vi "未命名 13.vi"() -> ()   [LabVIEW 2020]
uses:
  <vilib>/JDP Science/JSONtext/support/Format JSON Object.vi
  <vilib>/JDP Science/JSONtext/JSONtext.lvlib
panel:
  out "<JSON> 2":string[](array[string]) caption="<JSON>Elements"
  out "输出数组":string[](array[string])
  in  "数组":string[](array[string])
  in  "JSON Items":string[](array[string])
  in  "Item Names":string[](array[string])
  out "<JSON>":string caption="<JSON>Object"
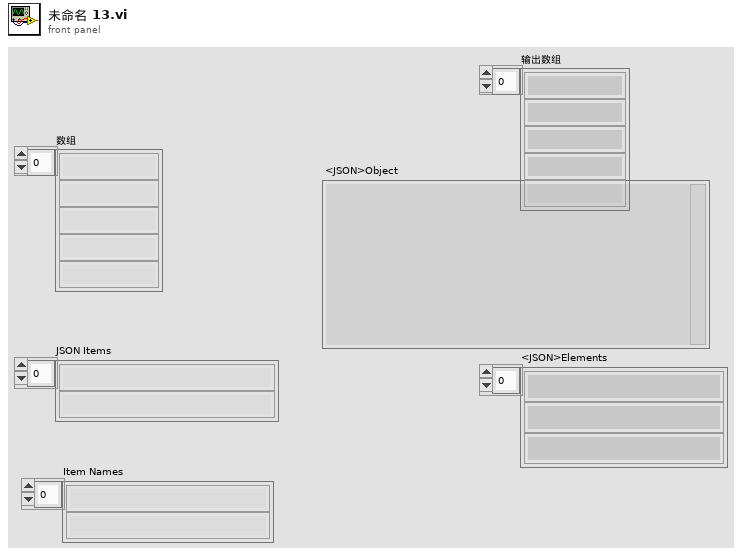
[diagram p1: front panel]
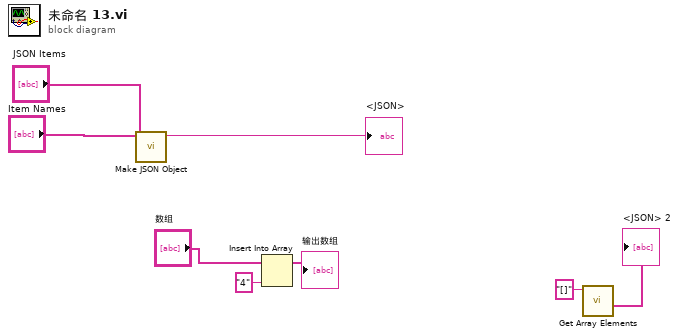
[diagram p0: block diagram]
diagram:
  n1 = call <vilib>:"Make JSON Object.vi"("JSON Items"="JSON Items", "Item Names"="Item Names") -> ("<JSON>"=→"<JSON>":string)  [unwired: 8 in, 1 out]
  n2 = Insert Into Array(array="数组", new element="4" ("新元素/子数组")) -> (→"输出数组":string[])  [unwired: 1 in]
  n3 = call <vilib>:"Get Array Elements.vi"("JSON"="[]") -> ("<JSON>"=→"<JSON> 2":string[])  [unwired: 8 in, 2 out]
